vi "DSF.Engine.Framework.Error Handler.Handle Transceiver Error.vi"(8 "error in (no error)":errorcluster, 10 "transceiver error":errorcluster, 11 "Framework in":refnum<class "DSF.Engine.Framework.lvclass">) -> (0 "error out":errorcluster, 3 "Framework out":refnum<class "DSF.Engine.Framework.lvclass">)   [LabVIEW 2017, in "DSF.Engine.lvlib" / "DSF.Engine.Framework.lvclass"]
uses:
  DSF.Engine.Framework.lvclass
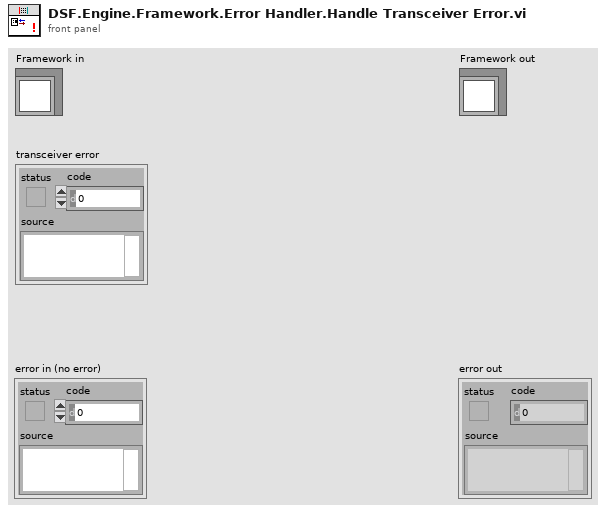
[diagram p1: front panel]
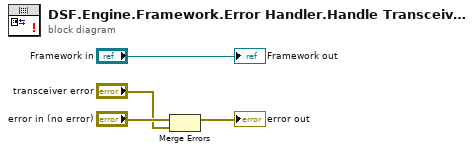
[diagram p0: block diagram]
diagram:
  n1 = Merge Errors("error in (no error)", "transceiver error") -> (→"error out":errorcluster)
  "Framework out" <- "Framework in"
